vi "ElevatorSafetyInterlocks.vi"(8 "Feed Forward Contribution":dbl, 9 "Elevator State In":string, 10 "Elevator Power In":dbl) -> (1 "Elevator State Out":string, 2 "Elevator Power Out":dbl)   [LabVIEW 2018]
uses:
  Inputs_DriverStation.vi
  SensorReadings.vi
  RobotStates.vi
panel:
  in  "Ignore Stall Safety (in)":dbl=85.0
  in  "Maximum (Climbing) Elevator Height (in)":dbl=65.0
  in  "Encoder Check Velocity (in/s)":dbl=0.1 format="%#_13g"
  in  "Maximum (Normal) Elevator Height (in)":dbl=92.0
  in  "Encoder Check Delay (ms)":u32=3000
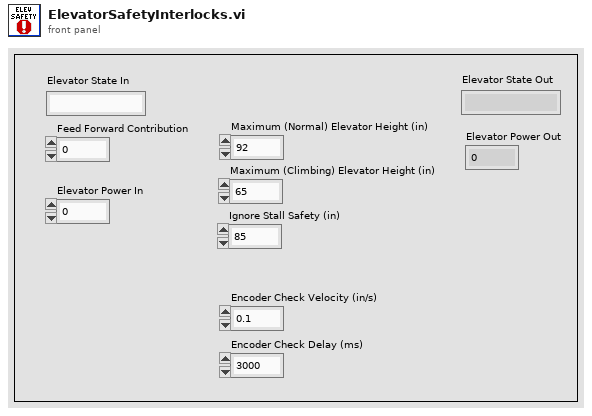
[diagram p1: front panel]
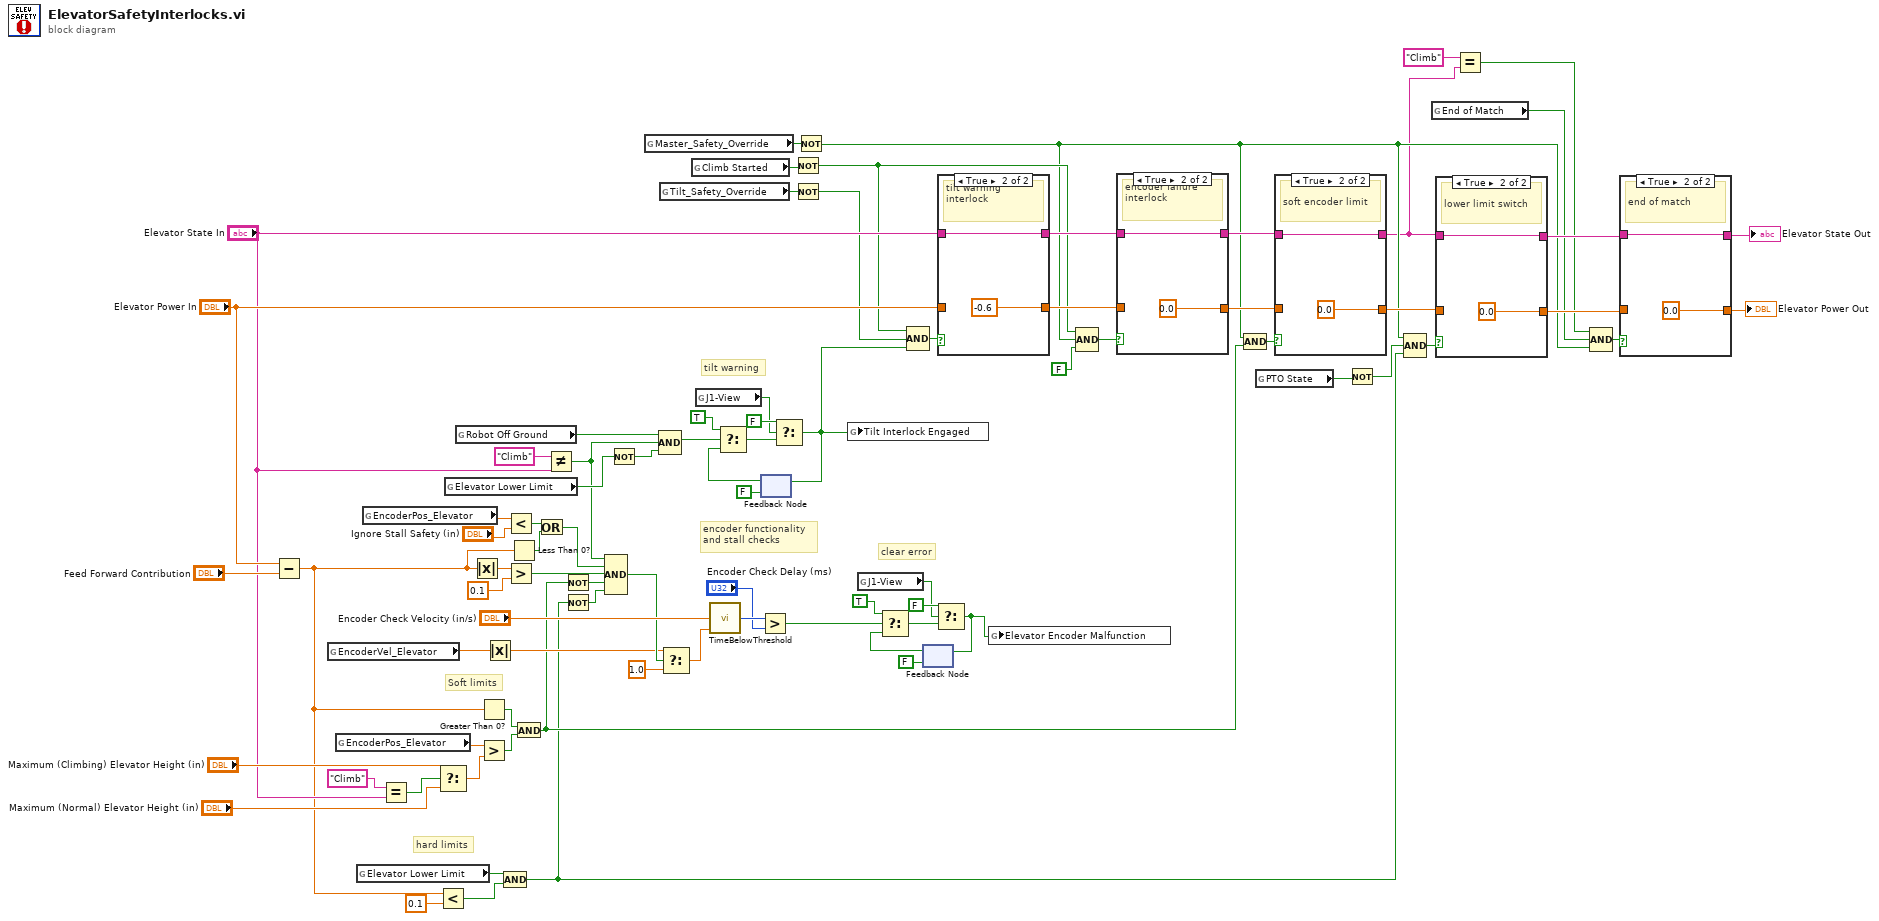
[diagram p0: block diagram]
diagram:
  # "clear error"
  # "tilt warning"
  # "hard limits"
  # "Soft limits"
  # "encoder functionality\nand stall checks"
  n1 = Subtract(x="Elevator Power In", y="Feed Forward Contribution") -> (x-y=w15:dbl)
  n2 = global read "SensorReadings.vi" "EncoderVel_Elevator"() -> (w82:dbl)
  n3 = global read "SensorReadings.vi" "EncoderPos_Elevator"() -> (w76:dbl)
  n4 = global read "SensorReadings.vi" "Elevator Lower Limit"() -> (w72:bool)
  n5 = global read "SensorReadings.vi" "EncoderPos_Elevator"() -> (w20:dbl)
  n6 = Equal?(x="Climb", y="Elevator State In") -> (x = y?=w41:bool)
  n7 = Select(t="Maximum (Climbing) Elevator Height (in)", s=w41, f="Maximum (Normal) Elevator Height (in)") -> (s? t:f=w47:dbl)
  n8 = Less?(x=w15, y=0.1) -> (x < y?=w57:bool)
  n9 = global read "SensorReadings.vi" "Elevator Lower Limit"() -> (w43:bool)
  n10 = global read "SensorReadings.vi" "Robot Off Ground"() -> (w44:bool)
  n11 = Absolute Value(x=w15) -> (abs(x)=w35:dbl)
  n12 = Greater Than 0?(x=w15) -> (x > 0?=w75:bool)
  n13 = Greater?(x=w76, y=w47) -> (0:w74:bool)
  n14 = Absolute Value(x=w82) -> (abs(x)=w27:dbl)
  n15 = Compound Arithmetic op=AND(w72, w57) -> (w21:bool)
  n16 = Less?(x=w20, y="Ignore Stall Safety (in)") -> (x < y?=w18:bool)
  n17 = Greater?(x=w35, y=0.1) -> (0:w31:bool)
  n18 = Less Than 0?(x=w15) -> (x < 0?=w16:bool)
  n19 = And(x=w75, y=w74) -> (x .and. y?=w23:bool)
  n20 = Or(x=w18, y=w16) -> (x .or. y?=w17:bool)
  n21 = Not Equal?(x="Climb", y="Elevator State In") -> (x != y?=w3:bool)
  n22 = Not(x=w23) -> (.not. x?=w30:bool)
  n23 = Not(x=w21) -> (.not. x?=w24:bool)
  n24 = Compound Arithmetic op=AND(w3, w17, w31, w30, w24) -> (w28:bool)
  n25 = Not(x=w43) -> (.not. x?=w38:bool)
  n26 = global read "Inputs_DriverStation.vi" "Master_Safety_Override"() -> (w83:bool)
  n27 = Compound Arithmetic op=AND(w44, w3, w38) -> (w61:bool)
  n28 = global read "Inputs_DriverStation.vi" "Tilt_Safety_Override"() -> (w2:bool)
  n29 = Select(t=w27, s=w28, f=1.0) -> (s? t:f=w29:dbl)
  n30 = global read "RobotStates.vi" "Climb Started"() -> (w46:bool)
  n31 = global read "Inputs_DriverStation.vi" "J1-View"() -> (w65:bool)
  n32 = call "TimeBelowThreshold.vi"("Current Value"=w29, "Threshold"="Encoder Check Velocity (in/s)") -> ("Time Below"=w79:u32)  [unwired: 3 in]
  n33 = Greater?(x=w79, y="Encoder Check Delay (ms)") -> (0:w33:bool)
  n34 = feedback #1(FALSE) -> (w69:bool)
  n35 = Select(t=TRUE, s=w61, f=w69) -> (s? t:f=w67:bool)
  n36 = Select(t=FALSE, s=w65, f=w67) -> (s? t:f=w37:bool)
  n37 = feedback-in #1(w37) -> ()
  n38 = Not(x=w46) -> (.not. x?=w39:bool)
  n39 = Not(x=w2) -> (.not. x?=w1:bool)
  n40 = Not(x=w83) -> (.not. x?=w8:bool)
  n41 = global write "RobotStates.vi" "Tilt Interlock Engaged"(w37) -> ()
  n42 = global read "Inputs_DriverStation.vi" "J1-View"() -> (w50:bool)
  n43 = Compound Arithmetic op=AND(w39, w1, w37) -> (w56:bool)
  n44 = feedback #2(FALSE) -> (w54:bool)
  n45 = Select(t=TRUE, s=w33, f=w54) -> (s? t:f=w52:bool)
  n46 = Select(t=FALSE, s=w50, f=w52) -> (s? t:f=w25:bool)
  n47 = feedback-in #2(w25) -> ()
  n48 = case shown="True" w56 {
    tunnel: [w84 -0.6 ("Elevator Power In")] -> w62
    tunnel: "Elevator State In" -> [w85 w86]
    tunnel: [w85 w86] -> w64
    tunnel: "Elevator Power In" -> [w84 _]
    frame False {
      # "tilt okay"
    }
    frame True {
      # "tilt warning interlock"
    }
  }
  n49 = global write "SensorReadings.vi" "Elevator Encoder Malfunction"(w25) -> ()
  n50 = Compound Arithmetic op=AND(w39, w8, FALSE) -> (w36:bool)
  n51 = case shown="True" w36 {
    tunnel: [w88 0.0 ("Elevator Power In")] -> w77
    tunnel: w62 -> [w88 _]
    tunnel: [w89 w91] -> w78
    tunnel: w64 -> [w89 w91]
    frame False {
      # "okay encoder"
    }
    frame True {
      # "encoder failure interlock"
    }
  }
  n52 = Compound Arithmetic op=AND(w8, w23) -> (w59:bool)
  n53 = global read "RobotStates.vi" "PTO State"() -> (w45:bool)
  n54 = case shown="True" w59 {
    tunnel: [w92 0.0 ("Elevator Power In")] -> w73
    tunnel: w77 -> [w92 _]
    tunnel: [w93 w95] -> w6
    tunnel: w78 -> [w93 w95]
    frame False {
      # "okay height"
    }
    frame True {
      # "soft encoder limit"
    }
  }
  n55 = Not(x=w45) -> (.not. x?=w22:bool)
  n56 = Compound Arithmetic op=AND(w8, w22, w21) -> (w58:bool)
  n57 = global read "RobotStates.vi" "End of Match"() -> (w5:bool)
  n58 = case shown="True" w58 {
    tunnel: [w96 0.0 ("Elevator Power In")] -> w12
    tunnel: w73 -> [w96 _]
    tunnel: [w97 w99] -> w13
    tunnel: w6 -> [w97 w99]
    frame False {
      # "okay lower limit switch"
    }
    frame True {
      # "lower limit switch"
    }
  }
  n59 = Equal?(x="Climb", y=w6) -> (x = y?=w4:bool)
  n60 = Compound Arithmetic op=AND(w4, w5, w8) -> (w9:bool)
  n61 = case shown="True" w9 {
    tunnel: [w100 0.0 ("Elevator Power In")] -> w10
    tunnel: w12 -> [w100 _]
    tunnel: [w101 w103] -> w11
    tunnel: w13 -> [w101 w103]
    frame False {
      # "not end of match"
    }
    frame True {
      # "end of match"
    }
  }
  "Elevator Power Out" <- w10
  "Elevator State Out" <- w11
